vi "CAN_READ_SK.vi"(0 "ID101":u8[](array[numeric]) format="%x", 5 "ID102":u8[](array[numeric]) format="%x", 7 "ID103":u8[](array[numeric]) format="%x", 9 "ID106":u8[](array[numeric]) format="%x", 11 "ID109":u8[](array[numeric]) format="%x") -> (4 "cluster de sortie":T1)   [LabVIEW 2020]
panel:
  in  "cluster input":T2
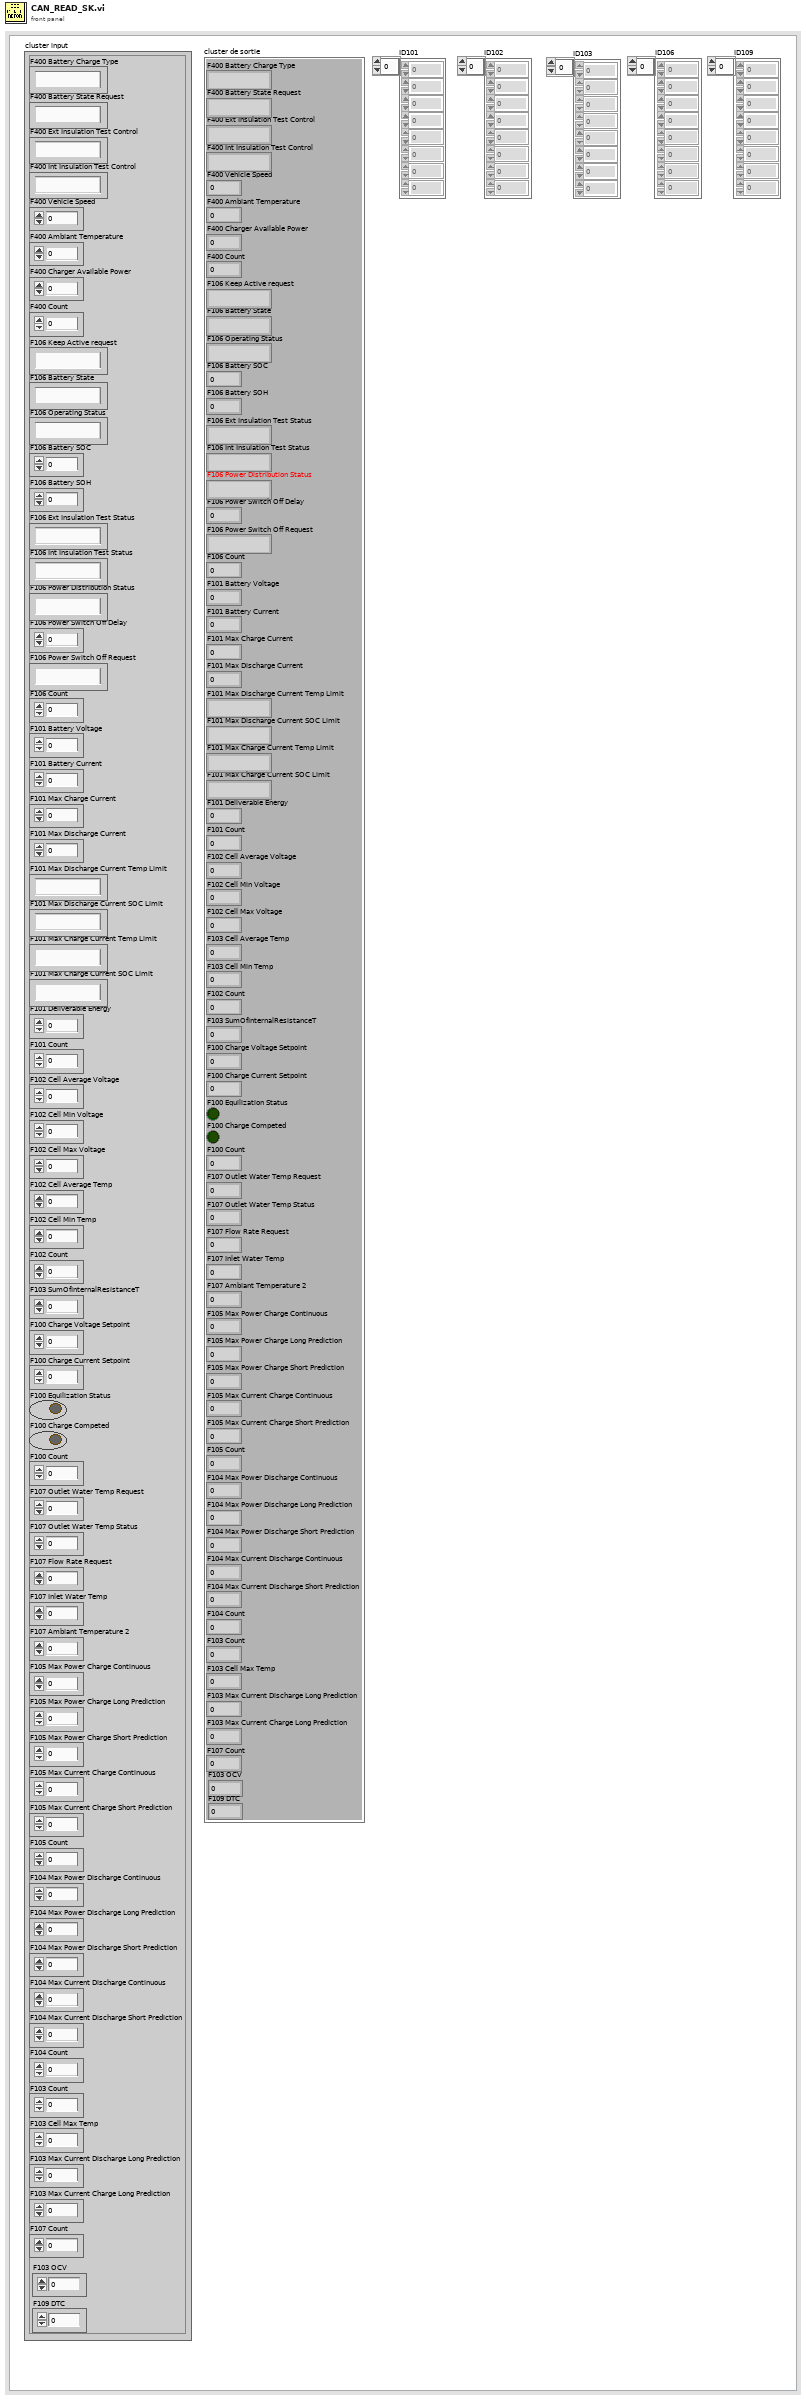
[diagram p1: front panel]
types:
  T1 = cluster{"F400 Battery Charge Type":string, "F400 Battery State Request":string, "F400 Ext Insulation Test Control":string, "F400 Int Insulation Test Control":string, "F400 Vehicle Speed":i32, "F400 Ambiant Temperature":i32, "F400 Charger Available Power":i32, "F400 Count":i32, "F106 Keep Active request":string, "F106 Battery State":string, "F106 Operating Status":string, "F106 Battery SOC":dbl, "F106 Battery SOH":dbl, "F106 Ext Insulation Test Status":string, "F106 Int Insulation Test Status":string, "F106 Power Distribution Status":string, "F106 Power Switch Off Delay":i32, "F106 Power Switch Off Request":string, "F106 Count":i32, "F101 Battery Voltage":u32, "F101 Battery Current":dbl, "F101 Max Charge Current":u32, "F101 Max Discharge Current":u32, "F101 Max Discharge Current Temp Limit":string, "F101 Max Discharge Current SOC Limit":string, "F101 Max Charge Current Temp Limit":string, "F101 Max Charge Current SOC Limit":string, "F101 Deliverable Energy":dbl, "F101 Count":u32, "F102 Cell Average Voltage":u32, "F102 Cell Min Voltage":u32, "F102 Cell Max Voltage":u32, "F103 Cell Average Temp":i32, "F103 Cell Min Temp":i32, "F102 Count":u32, "F103 SumOfInternalResistanceT":i32, "F100 Charge Voltage Setpoint":i32, "F100 Charge Current Setpoint":dbl, "F100 Equilization Status":bool, "F100 Charge Competed":bool, "F100 Count":i32, "F107 Outlet Water Temp Request":i32, "F107 Outlet Water Temp Status":i32, "F107 Flow Rate Request":i32, "F107 Inlet Water Temp":i32, "F107 Ambiant Temperature 2":i32, "F105 Max Power Charge Continuous":i32, "F105 Max Power Charge Long Prediction":i32, "F105 Max Power Charge Short Prediction":i32, "F105 Max Current Charge Continuous":i32, "F105 Max Current Charge Short Prediction":i32, "F105 Count ":i32, "F104 Max Power Discharge Continuous":i32, "F104 Max Power Discharge Long Prediction":i32, "F104 Max Power Discharge Short Prediction":i32, "F104 Max Current Discharge Continuous":i32, "F104 Max Current Discharge Short Prediction":i32, "F104 Count ":i32, "F103 Count":i32, "F103 Cell Max Temp":i32, "F103 Max Current Discharge Long Prediction":i32, "F103 Max Current Charge Long Prediction":i32, "F107 Count":i32, "F103 OCV":i32, "F109 DTC":i32}
  T2 = cluster{"F400 Battery Charge Type":string, "F400 Battery State Request":string, "F400 Ext Insulation Test Control":string, "F400 Int Insulation Test Control":string, "F400 Vehicle Speed":i32, "F400 Ambiant Temperature":i32, "F400 Charger Available Power":i32, "F400 Count":i32, "F106 Keep Active request":string, "F106 Battery State":string, "F106 Operating Status":string, "F106 Battery SOC":dbl, "F106 Battery SOH":dbl, "F106 Ext Insulation Test Status":string, "F106 Int Insulation Test Status":string, "F106 Power Distribution Status":string, "F106 Power Switch Off Delay":i32, "F106 Power Switch Off Request":string, "F106 Count":i32, "F101 Battery Voltage":u32, "F101 Battery Current":dbl, "F101 Max Charge Current":u32, "F101 Max Discharge Current":u32, "F101 Max Discharge Current Temp Limit":string, "F101 Max Discharge Current SOC Limit":string, "F101 Max Charge Current Temp Limit":string, "F101 Max Charge Current SOC Limit":string, "F101 Deliverable Energy":dbl, "F101 Count":u32, "F102 Cell Average Voltage":u32, "F102 Cell Min Voltage":u32, "F102 Cell Max Voltage":u32, "F102 Cell Average Temp":i32, "F102 Cell Min Temp":i32, "F102 Count":u32, "F103 SumOfInternalResistanceT":i32, "F100 Charge Voltage Setpoint":i32, "F100 Charge Current Setpoint":dbl, "F100 Equilization Status":bool, "F100 Charge Competed":bool, "F100 Count":i32, "F107 Outlet Water Temp Request":i32, "F107 Outlet Water Temp Status":i32, "F107 Flow Rate Request":i32, "F107 Inlet Water Temp":i32, "F107 Ambiant Temperature 2":i32, "F105 Max Power Charge Continuous":i32, "F105 Max Power Charge Long Prediction":i32, "F105 Max Power Charge Short Prediction":i32, "F105 Max Current Charge Continuous":i32, "F105 Max Current Charge Short Prediction":i32, "F105 Count ":i32, "F104 Max Power Discharge Continuous":i32, "F104 Max Power Discharge Long Prediction":i32, "F104 Max Power Discharge Short Prediction":i32, "F104 Max Current Discharge Continuous":i32, "F104 Max Current Discharge Short Prediction":i32, "F104 Count ":i32, "F103 Count":i32, "F103 Cell Max Temp":i32, "F103 Max Current Discharge Long Prediction":i32, "F103 Max Current Charge Long Prediction":i32, "F107 Count":i32, "F103 OCV":i32, "F109 DTC":i32}
  T3 = cluster{"ID103[0]":u8, "ID103[1]":u8, "ID103[2]":u8, "ID103[3]":u8, "ID103[4]":u8, "ID103[5]":u8, "ID103[6]":u8, "ID103[7]":u8}
  T4 = cluster{"ID102[0]":u8, "ID102[1]":u8, "ID102[2]":u8, "ID102[3]":u8, "ID102[4]":u8, "ID102[5]":u8, "ID102[6]":u8, "ID102[7]":u8}
  T5 = cluster{"ID101[0]":u8, "ID101[1]":u8, "ID101[2]":u8, "ID101[3]":u8, "ID101[4]":u8, "ID101[5]":u8, "ID101[6]":u8, "ID101[7]":u8}
  T6 = cluster{"ID106[0]":u8, "ID106[1]":u8, "ID106[2]":u8, "ID106[3]":u8, "ID106[4]":u8, "ID106[5]":u8, "ID106[6]":u8, "ID106[7]":u8}
  T7 = cluster{"ID109[0]":u8, "ID109[1]":u8, "ID109[2]":u8, "ID109[3]":u8, "ID109[4]":u8, "ID109[5]":u8, "ID109[6]":u8, "ID109[7]":u8}
  T8 = cluster{"Boolean array[0]":bool, "Boolean array[1]":bool, "Boolean array[2]":bool, "Boolean array[3]":bool, "Boolean array[4]":bool, "Boolean array[5]":bool, "Boolean array[6]":bool, "Boolean array[7]":bool}
  T9 = cluster{"Boolean array[0]":bool, "Boolean array[1]":bool}
  T10 = cluster{"Boolean array[3]":bool, "Boolean array[4]":bool, "Boolean array[5]":bool}
  T11 = cluster{"Boolean array[2]":bool, "Boolean array[3]":bool, "Boolean array[4]":bool}
  T12 = cluster{"Boolean array[6]":bool, "Boolean array[7]":bool, "Boolean array[0]":bool, "Boolean array[1]":bool, "Boolean array[2]":bool, "Boolean array[3]":bool, "Boolean array[4]":bool, "Boolean array[5]":bool, "Boolean array[6]":bool, "Boolean array[7]":bool}
  T13 = cluster{"Boolean array[7]":bool, "Boolean array[6]":bool, "Boolean array[0]":bool, "Boolean array[1]":bool, "Boolean array[2]":bool, "Boolean array[3]":bool, "Boolean array[4]":bool, "Boolean array[5]":bool, "Boolean array[6]":bool, "Boolean array[7]":bool}
  T14 = cluster{"Boolean array[6]":bool, "Boolean array[7]":bool, "Boolean array[0]":bool, "Boolean array[1]":bool, "Boolean array[2]":bool, "Boolean array[3]":bool, "Boolean array[4]":bool, "Boolean array[5]":bool, "Boolean array[6]":bool, "Boolean array[7]":bool, "Boolean array[0]":bool, "Boolean array[1]":bool, "Boolean array[2]":bool}
  T15 = cluster{"Boolean array[0]":bool, "Boolean array[1]":bool, "Boolean array[2]":bool, "Boolean array[3]":bool, "Boolean array[4]":bool, "Boolean array[5]":bool, "Boolean array[6]":bool, "Boolean array[7]":bool, "Boolean array[0]":bool, "Boolean array[1]":bool, "Boolean array[2]":bool, "Boolean array[3]":bool, "Boolean array[4]":bool, "Boolean array[5]":bool}
  T16 = cluster{"Boolean array[1]":bool, "Boolean array[2]":bool, "Boolean array[3]":bool, "Boolean array[4]":bool, "Boolean array[5]":bool, "Boolean array[6]":bool, "Boolean array[7]":bool, "Boolean array[0]":bool, "Boolean array[1]":bool, "Boolean array[2]":bool, "Boolean array[3]":bool, "Boolean array[4]":bool, "Boolean array[5]":bool}
  T17 = cluster{"Boolean array[3]":bool, "Boolean array[4]":bool, "Boolean array[5]":bool, "Boolean array[6]":bool, "Boolean array[7]":bool, "Boolean array[0]":bool, "Boolean array[1]":bool, "Boolean array[2]":bool, "Boolean array[3]":bool, "Boolean array[4]":bool, "Boolean array[5]":bool, "Boolean array[6]":bool, "Boolean array[7]":bool}
  T18 = cluster{"Boolean array[0]":bool, "Boolean array[1]":bool, "Boolean array[2]":bool, "Boolean array[3]":bool, "Boolean array[4]":bool, "Boolean array[5]":bool, "Boolean array[6]":bool, "Boolean array[7]":bool, "Boolean array[0]":bool, "Boolean array[1]":bool, "Boolean array[2]":bool, "Boolean array[3]":bool, "Boolean array[4]":bool, "Boolean array[5]":bool, "Boolean array[6]":bool, "Boolean array[7]":bool, "Boolean array[0]":bool, "Boolean array[1]":bool, "Boolean array[2]":bool, "Boolean array[3]":bool, "Boolean array[4]":bool, "Boolean array[5]":bool, "Boolean array[6]":bool, "Boolean array[7]":bool}
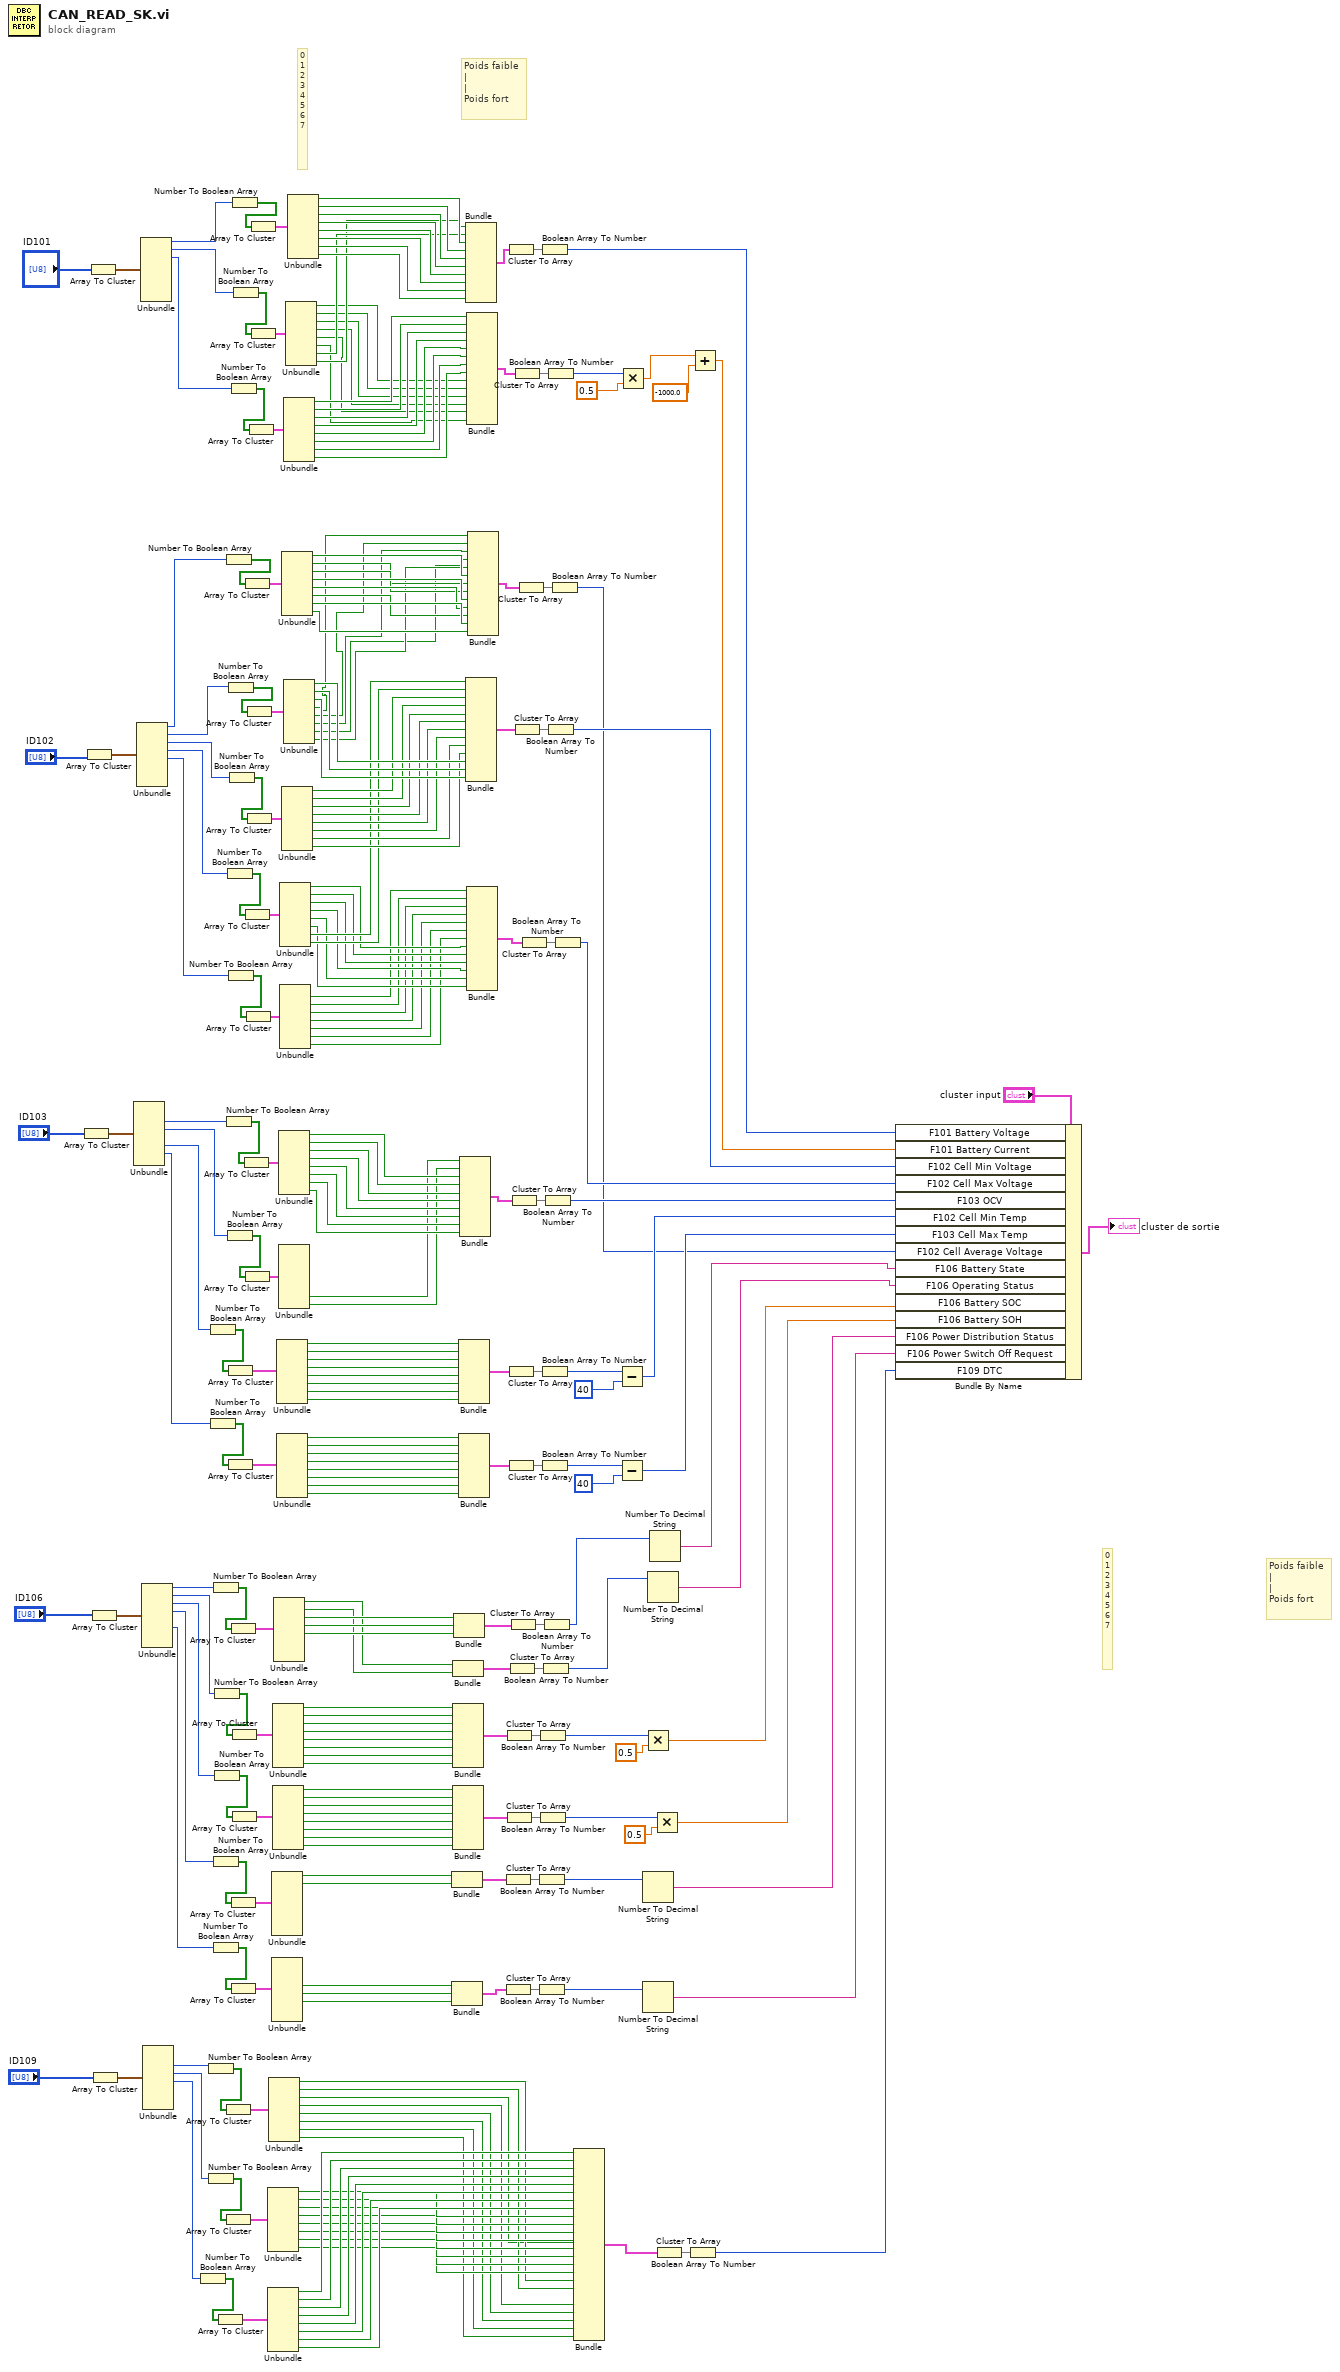
[diagram p0: block diagram]
diagram:
  # "Poids faible\n|\n|\nPoids fort"
  # "0\n1\n2\n3\n4\n5\n6\n7"
  # "Poids faible\n|\n|\nPoids fort"
  # "0\n1\n2\n3\n4\n5\n6\n7"
  n1 = Array To Cluster(array="ID103") -> (cluster=w180:T3)
  n2 = Array To Cluster(array="ID102") -> (cluster=w222:T4)
  n3 = Array To Cluster(array="ID101") -> (cluster=w259:T5)
  n4 = Array To Cluster(array="ID106") -> (cluster=w143:T6)
  n5 = Array To Cluster(array="ID109") -> (cluster=w84:T7)
  n6 = Unbundle(w180) -> ("ID103[2]"=w174:u8, "ID103[3]"=w165:u8, "ID103[5]"=w157:u8, "ID103[6]"=w31:u8)  [unwired: 4 out]
  n7 = Unbundle(w222) -> ("ID102[0]"=w17:u8, "ID102[1]"=w205:u8, "ID102[2]"=w204:u8, "ID102[3]"=w203:u8, "ID102[4]"=w202:u8)  [unwired: 3 out]
  n8 = Unbundle(w259) -> ("ID101[0]"=w263:u8, "ID101[1]"=w264:u8, "ID101[2]"=w248:u8)  [unwired: 5 out]
  n9 = Unbundle(w143) -> ("ID106[0]"=w139:u8, "ID106[1]"=w125:u8, "ID106[2]"=w102:u8, "ID106[3]"=w95:u8, "ID106[5]"=w89:u8)  [unwired: 3 out]
  n10 = Unbundle(w84) -> ("ID109[2]"=w81:u8, "ID109[3]"=w78:u8, "ID109[4]"=w77:u8)  [unwired: 5 out]
  n11 = Number To Boolean Array(number=w77) -> (Boolean array=w79:bool[])
  n12 = Number To Boolean Array(number=w81) -> (Boolean array=w82:bool[])
  n13 = Number To Boolean Array(number=w78) -> (Boolean array=w80:bool[])
  n14 = Number To Boolean Array(number=w157) -> (Boolean array=w159:bool[])
  n15 = Number To Boolean Array(number=w31) -> (Boolean array=w32:bool[])
  n16 = Number To Boolean Array(number=w139) -> (Boolean array=w140:bool[])
  n17 = Number To Boolean Array(number=w95) -> (Boolean array=w101:bool[])
  n18 = Number To Boolean Array(number=w89) -> (Boolean array=w90:bool[])
  n19 = Number To Boolean Array(number=w125) -> (Boolean array=w127:bool[])
  n20 = Number To Boolean Array(number=w102) -> (Boolean array=w103:bool[])
  n21 = Array To Cluster(array=w79) -> (cluster=w74:T8)
  n22 = Array To Cluster(array=w82) -> (cluster=w76:T8)
  n23 = Array To Cluster(array=w80) -> (cluster=w75:T8)
  n24 = Number To Boolean Array(number=w17) -> (Boolean array=w19:bool[])
  n25 = Number To Boolean Array(number=w174) -> (Boolean array=w175:bool[])
  n26 = Number To Boolean Array(number=w203) -> (Boolean array=w226:bool[])
  n27 = Number To Boolean Array(number=w165) -> (Boolean array=w178:bool[])
  n28 = Array To Cluster(array=w159) -> (cluster=w158:T8)
  n29 = Array To Cluster(array=w32) -> (cluster=w33:T8)
  n30 = Number To Boolean Array(number=w205) -> (Boolean array=w220:bool[])
  n31 = Number To Boolean Array(number=w202) -> (Boolean array=w197:bool[])
  n32 = Number To Boolean Array(number=w204) -> (Boolean array=w223:bool[])
  n33 = Array To Cluster(array=w140) -> (cluster=w141:T8)
  n34 = Array To Cluster(array=w101) -> (cluster=w100:T8)
  n35 = Array To Cluster(array=w90) -> (cluster=w91:T8)
  n36 = Number To Boolean Array(number=w248) -> (Boolean array=w249:bool[])
  n37 = Array To Cluster(array=w127) -> (cluster=w126:T8)
  n38 = Array To Cluster(array=w103) -> (cluster=w104:T8)
  n39 = Number To Boolean Array(number=w263) -> (Boolean array=w262:bool[])
  n40 = Number To Boolean Array(number=w264) -> (Boolean array=w256:bool[])
  n41 = Array To Cluster(array=w175) -> (cluster=w176:T8)
  n42 = Array To Cluster(array=w19) -> (cluster=w18:T8)
  n43 = Array To Cluster(array=w226) -> (cluster=w225:T8)
  n44 = Array To Cluster(array=w178) -> (cluster=w177:T8)
  n45 = Array To Cluster(array=w197) -> (cluster=w198:T8)
  n46 = Array To Cluster(array=w220) -> (cluster=w221:T8)
  n47 = Array To Cluster(array=w223) -> (cluster=w224:T8)
  n48 = Array To Cluster(array=w249) -> (cluster=w250:T8)
  n49 = Array To Cluster(array=w262) -> (cluster=w261:T8)
  n50 = Array To Cluster(array=w256) -> (cluster=w255:T8)
  n51 = Unbundle(w75) -> ("Boolean array[0]"=w65:bool, "Boolean array[1]"=w64:bool, "Boolean array[2]"=w63:bool, "Boolean array[3]"=w62:bool, "Boolean array[4]"=w61:bool, "Boolean array[5]"=w60:bool, "Boolean array[6]"=w59:bool, "Boolean array[7]"=w58:bool)
  n52 = Unbundle(w74) -> ("Boolean array[0]"=w73:bool, "Boolean array[1]"=w72:bool, "Boolean array[2]"=w71:bool, "Boolean array[3]"=w70:bool, "Boolean array[4]"=w69:bool, "Boolean array[5]"=w68:bool, "Boolean array[6]"=w67:bool, "Boolean array[7]"=w66:bool)
  n53 = Unbundle(w76) -> ("Boolean array[0]"=w57:bool, "Boolean array[1]"=w56:bool, "Boolean array[2]"=w55:bool, "Boolean array[3]"=w54:bool, "Boolean array[4]"=w53:bool, "Boolean array[5]"=w52:bool, "Boolean array[6]"=w51:bool, "Boolean array[7]"=w50:bool)
  n54 = Unbundle(w100) -> ("Boolean array[0]"=w99:bool, "Boolean array[1]"=w98:bool)  [unwired: 6 out]
  n55 = Unbundle(w91) -> ("Boolean array[3]"=w88:bool, "Boolean array[4]"=w87:bool, "Boolean array[5]"=w86:bool)  [unwired: 5 out]
  n56 = Unbundle(w126) -> ("Boolean array[0]"=w124:bool, "Boolean array[1]"=w123:bool, "Boolean array[2]"=w122:bool, "Boolean array[3]"=w121:bool, "Boolean array[4]"=w120:bool, "Boolean array[5]"=w119:bool, "Boolean array[6]"=w118:bool, "Boolean array[7]"=w117:bool)
  n57 = Unbundle(w104) -> ("Boolean array[0]"=w105:bool, "Boolean array[1]"=w106:bool, "Boolean array[2]"=w107:bool, "Boolean array[3]"=w108:bool, "Boolean array[4]"=w109:bool, "Boolean array[5]"=w110:bool, "Boolean array[6]"=w111:bool, "Boolean array[7]"=w112:bool)
  n58 = Unbundle(w141) -> ("Boolean array[0]"=w132:bool, "Boolean array[1]"=w131:bool, "Boolean array[2]"=w138:bool, "Boolean array[3]"=w137:bool, "Boolean array[4]"=w136:bool)  [unwired: 3 out]
  n59 = Unbundle(w158) -> ("Boolean array[0]"=w149:bool, "Boolean array[1]"=w150:bool, "Boolean array[2]"=w151:bool, "Boolean array[3]"=w152:bool, "Boolean array[4]"=w153:bool, "Boolean array[5]"=w154:bool, "Boolean array[6]"=w155:bool, "Boolean array[7]"=w156:bool)
  n60 = Unbundle(w33) -> ("Boolean array[0]"=w41:bool, "Boolean array[1]"=w40:bool, "Boolean array[2]"=w39:bool, "Boolean array[3]"=w38:bool, "Boolean array[4]"=w37:bool, "Boolean array[5]"=w36:bool, "Boolean array[6]"=w35:bool, "Boolean array[7]"=w34:bool)
  n61 = Unbundle(w176) -> ("Boolean array[0]"=w166:bool, "Boolean array[1]"=w167:bool, "Boolean array[2]"=w168:bool, "Boolean array[3]"=w169:bool, "Boolean array[4]"=w170:bool, "Boolean array[5]"=w171:bool, "Boolean array[6]"=w172:bool, "Boolean array[7]"=w173:bool)
  n62 = Unbundle(w177) -> ("Boolean array[6]"=w163:bool, "Boolean array[7]"=w164:bool)  [unwired: 6 out]
  n63 = Unbundle(w225) -> ("Boolean array[0]"=w191:bool, "Boolean array[1]"=w192:bool, "Boolean array[2]"=w193:bool, "Boolean array[3]"=w194:bool, "Boolean array[4]"=w195:bool, "Boolean array[5]"=w196:bool, "Boolean array[6]"=w206:bool, "Boolean array[7]"=w207:bool)
  n64 = Unbundle(w198) -> ("Boolean array[1]"=w181:bool, "Boolean array[2]"=w185:bool, "Boolean array[3]"=w186:bool, "Boolean array[4]"=w187:bool, "Boolean array[5]"=w188:bool, "Boolean array[6]"=w189:bool, "Boolean array[7]"=w190:bool)  [unwired: 1 out]
  n65 = Unbundle(w18) -> ("Boolean array[0]"=w9:bool, "Boolean array[1]"=w10:bool, "Boolean array[2]"=w11:bool, "Boolean array[3]"=w12:bool, "Boolean array[4]"=w13:bool, "Boolean array[5]"=w14:bool, "Boolean array[6]"=w15:bool, "Boolean array[7]"=w16:bool)
  n66 = Unbundle(w224) -> ("Boolean array[0]"=w208:bool, "Boolean array[1]"=w209:bool, "Boolean array[2]"=w210:bool, "Boolean array[3]"=w211:bool, "Boolean array[4]"=w212:bool, "Boolean array[5]"=w213:bool, "Boolean array[6]"=w214:bool, "Boolean array[7]"=w215:bool)
  n67 = Unbundle(w250) -> ("Boolean array[0]"=w247:bool, "Boolean array[1]"=w246:bool, "Boolean array[2]"=w245:bool, "Boolean array[3]"=w244:bool, "Boolean array[4]"=w243:bool, "Boolean array[5]"=w242:bool, "Boolean array[6]"=w241:bool, "Boolean array[7]"=w240:bool)
  n68 = Unbundle(w221) -> ("Boolean array[0]"=w216:bool, "Boolean array[1]"=w217:bool, "Boolean array[2]"=w218:bool, "Boolean array[3]"=w4:bool, "Boolean array[4]"=w5:bool, "Boolean array[5]"=w6:bool, "Boolean array[6]"=w7:bool, "Boolean array[7]"=w8:bool)
  n69 = Unbundle(w255) -> ("Boolean array[0]"=w239:bool, "Boolean array[1]"=w238:bool, "Boolean array[2]"=w237:bool, "Boolean array[3]"=w236:bool, "Boolean array[4]"=w235:bool, "Boolean array[5]"=w234:bool, "Boolean array[6]"=w254:bool, "Boolean array[7]"=w253:bool)
  n70 = Unbundle(w261) -> ("Boolean array[0]"=w265:bool, "Boolean array[1]"=w266:bool, "Boolean array[2]"=w272:bool, "Boolean array[3]"=w271:bool, "Boolean array[4]"=w270:bool, "Boolean array[5]"=w269:bool, "Boolean array[6]"=w268:bool, "Boolean array[7]"=w267:bool)
  n71 = Bundle("Boolean array[0]"=w99, "Boolean array[1]"=w98) -> (w96:T9)  [unwired: 1 in]
  n72 = Bundle("Boolean array[3]"=w88, "Boolean array[4]"=w87, "Boolean array[5]"=w86) -> (w93:T10)  [unwired: 1 in]
  n73 = Bundle("Boolean array[0]"=w132, "Boolean array[1]"=w131) -> (w129:T9)  [unwired: 1 in]
  n74 = Bundle("Boolean array[0]"=w124, "Boolean array[1]"=w123, "Boolean array[2]"=w122, "Boolean array[3]"=w121, "Boolean array[4]"=w120, "Boolean array[5]"=w119, "Boolean array[6]"=w118, "Boolean array[7]"=w117) -> (w115:T8)  [unwired: 1 in]
  n75 = Bundle("Boolean array[0]"=w105, "Boolean array[1]"=w106, "Boolean array[2]"=w107, "Boolean array[3]"=w108, "Boolean array[4]"=w109, "Boolean array[5]"=w110, "Boolean array[6]"=w111, "Boolean array[7]"=w112) -> (w114:T8)  [unwired: 1 in]
  n76 = Bundle("Boolean array[2]"=w138, "Boolean array[3]"=w137, "Boolean array[4]"=w136) -> (w134:T11)  [unwired: 1 in]
  n77 = Bundle("Boolean array[0]"=w149, "Boolean array[1]"=w150, "Boolean array[2]"=w151, "Boolean array[3]"=w152, "Boolean array[4]"=w153, "Boolean array[5]"=w154, "Boolean array[6]"=w155, "Boolean array[7]"=w156) -> (w147:T8)  [unwired: 1 in]
  n78 = Bundle("Boolean array[0]"=w41, "Boolean array[1]"=w40, "Boolean array[2]"=w39, "Boolean array[3]"=w38, "Boolean array[4]"=w37, "Boolean array[5]"=w36, "Boolean array[6]"=w35, "Boolean array[7]"=w34) -> (w43:T8)  [unwired: 1 in]
  n79 = Bundle("Boolean array[6]"=w163, "Boolean array[7]"=w164, "Boolean array[0]"=w166, "Boolean array[1]"=w167, "Boolean array[2]"=w168, "Boolean array[3]"=w169, "Boolean array[4]"=w170, "Boolean array[5]"=w171, "Boolean array[6]"=w172, "Boolean array[7]"=w173) -> (w161:T12)  [unwired: 1 in]
  n80 = Bundle("Boolean array[7]"=w253, "Boolean array[6]"=w254, "Boolean array[0]"=w265, "Boolean array[1]"=w266, "Boolean array[2]"=w272, "Boolean array[3]"=w271, "Boolean array[4]"=w270, "Boolean array[5]"=w269, "Boolean array[6]"=w268, "Boolean array[7]"=w267) -> (w252:T13)  [unwired: 1 in]
  n81 = Bundle("Boolean array[6]"=w206, "Boolean array[7]"=w207, "Boolean array[0]"=w208, "Boolean array[1]"=w209, "Boolean array[2]"=w210, "Boolean array[3]"=w211, "Boolean array[4]"=w212, "Boolean array[5]"=w213, "Boolean array[6]"=w214, "Boolean array[7]"=w215, "Boolean array[0]"=w216, "Boolean array[1]"=w217, "Boolean array[2]"=w218) -> (w200:T14)  [unwired: 1 in]
  n82 = Bundle("Boolean array[0]"=w247, "Boolean array[1]"=w246, "Boolean array[2]"=w245, "Boolean array[3]"=w244, "Boolean array[4]"=w243, "Boolean array[5]"=w242, "Boolean array[6]"=w241, "Boolean array[7]"=w240, "Boolean array[0]"=w239, "Boolean array[1]"=w238, "Boolean array[2]"=w237, "Boolean array[3]"=w236, "Boolean array[4]"=w235, "Boolean array[5]"=w234) -> (w233:T15)  [unwired: 1 in]
  n83 = Bundle("Boolean array[1]"=w181, "Boolean array[2]"=w185, "Boolean array[3]"=w186, "Boolean array[4]"=w187, "Boolean array[5]"=w188, "Boolean array[6]"=w189, "Boolean array[7]"=w190, "Boolean array[0]"=w191, "Boolean array[1]"=w192, "Boolean array[2]"=w193, "Boolean array[3]"=w194, "Boolean array[4]"=w195, "Boolean array[5]"=w196) -> (w183:T16)  [unwired: 1 in]
  n84 = Bundle("Boolean array[3]"=w4, "Boolean array[4]"=w5, "Boolean array[5]"=w6, "Boolean array[6]"=w7, "Boolean array[7]"=w8, "Boolean array[0]"=w9, "Boolean array[1]"=w10, "Boolean array[2]"=w11, "Boolean array[3]"=w12, "Boolean array[4]"=w13, "Boolean array[5]"=w14, "Boolean array[6]"=w15, "Boolean array[7]"=w16) -> (w2:T17)  [unwired: 1 in]
  n85 = Cluster To Array(cluster=w96) -> (array=w97:bool[])
  n86 = Cluster To Array(cluster=w93) -> (array=w92:bool[])
  n87 = Cluster To Array(cluster=w115) -> (array=w116:bool[])
  n88 = Cluster To Array(cluster=w114) -> (array=w113:bool[])
  n89 = Cluster To Array(cluster=w252) -> (array=w251:bool[])
  n90 = Cluster To Array(cluster=w147) -> (array=w148:bool[])
  n91 = Cluster To Array(cluster=w43) -> (array=w42:bool[])
  n92 = Cluster To Array(cluster=w129) -> (array=w130:bool[])
  n93 = Cluster To Array(cluster=w134) -> (array=w135:bool[])
  n94 = Cluster To Array(cluster=w161) -> (array=w162:bool[])
  n95 = Cluster To Array(cluster=w233) -> (array=w232:bool[])
  n96 = Cluster To Array(cluster=w200) -> (array=w201:bool[])
  n97 = Cluster To Array(cluster=w2) -> (array=w3:bool[])
  n98 = Cluster To Array(cluster=w183) -> (array=w184:bool[])
  n99 = Boolean Array To Number(Boolean array=w97) -> (number=w94:u32)
  n100 = Boolean Array To Number(Boolean array=w92) -> (number=w85:u32)
  n101 = Boolean Array To Number(Boolean array=w116) -> (number=w21:u32)
  n102 = Boolean Array To Number(Boolean array=w113) -> (number=w46:u32)
  n103 = Boolean Array To Number(Boolean array=w251) -> (number=w258:u32)
  n104 = Boolean Array To Number(Boolean array=w148) -> (number=w144:u32)
  n105 = Boolean Array To Number(Boolean array=w42) -> (number=w45:u32)
  n106 = Boolean Array To Number(Boolean array=w130) -> (number=w128:u32)
  n107 = Boolean Array To Number(Boolean array=w135) -> (number=w133:u32)
  n108 = Boolean Array To Number(Boolean array=w162) -> (number=w160:u32)
  n109 = Boolean Array To Number(Boolean array=w232) -> (number=w230:u32)
  n110 = Boolean Array To Number(Boolean array=w201) -> (number=w199:u32)
  n111 = Boolean Array To Number(Boolean array=w3) -> (number=w1:u32)
  n112 = Boolean Array To Number(Boolean array=w184) -> (number=w182:u32)
  n113 = Bundle("Boolean array[0]"=w73, "Boolean array[1]"=w72, "Boolean array[2]"=w71, "Boolean array[3]"=w70, "Boolean array[4]"=w69, "Boolean array[5]"=w68, "Boolean array[6]"=w67, "Boolean array[7]"=w66, "Boolean array[0]"=w65, "Boolean array[1]"=w64, "Boolean array[2]"=w63, "Boolean array[3]"=w62, "Boolean array[4]"=w61, "Boolean array[5]"=w60, "Boolean array[6]"=w59, "Boolean array[7]"=w58, "Boolean array[0]"=w57, "Boolean array[1]"=w56, "Boolean array[2]"=w55, "Boolean array[3]"=w54, "Boolean array[4]"=w53, "Boolean array[5]"=w52, "Boolean array[6]"=w51, "Boolean array[7]"=w50) -> (w48:T18)  [unwired: 1 in]
  n114 = Subtract(x=w144, y=u32 40) -> (x-y=w145:u32)
  n115 = Subtract(x=w45, y=u32 40) -> (x-y=w24:u32)
  n116 = Multiply(x=w230, y=0.5) -> (x*y=w229:dbl)
  n117 = Multiply(x=w21, y=0.5) -> (x*y=w20:dbl)
  n118 = Number To Decimal String(number=w94) -> (decimal integer string=w28:string)  [unwired: 1 in]
  n119 = Number To Decimal String(number=w85) -> (decimal integer string=w29:string)  [unwired: 1 in]
  n120 = Number To Decimal String(number=w128) -> (decimal integer string=w26:string)  [unwired: 1 in]
  n121 = Number To Decimal String(number=w133) -> (decimal integer string=w25:string)  [unwired: 1 in]
  n122 = Multiply(x=w46, y=0.5) -> (x*y=w27:dbl)
  n123 = Cluster To Array(cluster=w48) -> (array=w49:bool[])
  n124 = Boolean Array To Number(Boolean array=w49) -> (number=w30:u32)
  n125 = Add(x=w229, y=-1000.0) -> (x+y=w227:dbl)
  n126 = Bundle By Name(cluster="cluster input", "F101 Battery Voltage"=w258, "F101 Battery Current"=w227, "F102 Cell Min Voltage"=w199, "F102 Cell Max Voltage"=w182, "F103 OCV"=w160, "F102 Cell Min Temp"=w145, "F103 Cell Max Temp"=w24, "F102 Cell Average Voltage"=w1, "F106 Battery State"=w25, "F106 Operating Status"=w26, "F106 Battery SOC"=w20, "F106 Battery SOH"=w27, "F106 Power Distribution Status"=w28, "F106 Power Switch Off Request"=w29, "F109 DTC"=w30) -> (→"cluster de sortie":T2)
